vi "GUI_LPG-VikynoRV125.vi"() -> ()   [LabVIEW 2020]
uses:
  <vilib>/Instr/_visa.llb/VISA Configure Serial Port (Instr).vi
panel:
  out "Gen Torque (N.m)":sgl format="%#_6f"
  out "Engine Speed (RPM)":sgl(knob) scale=0.0..2500.0
  out "Average MAF Value (g/s)":dbl format="%.2f"
  in  "Reset Torque":bool
  out "MAF (g/s)":dbl format="%.2f"
  in  "Diesel Used (g)":dbl
  in  "LPG  Consumed (g)":dbl
  out "Engine Torque (N.m)":dbl format="%#_4f"
  out "Equivalent Ratio (Phi)":dbl format="%.2f"
  out "Engine Power (kW)":dbl
  in  "Tab Control":enum32{"PID", "Error"}(tab)
  out "PID Engine Speed Graph":cluster{sgl, "Set Engine Speed":sgl}(graph)
  out "Actual Engine Speed (RPM)":sgl
  out "error out":errorcluster
  out "error out 2":errorcluster
  in  "Stop":bool
  in  "Number of sample":u16=50
  out "?":bool
  out "?":bool
  in  "Arduino UNO port":refnum<visa-resource-name>="COM8"
  in  "Loop Time (ms)":u32=25
  in  "ESP32 port":refnum<visa-resource-name>="COM9"
  in  "INJT 2 (CA)":sgl=10.0 min=0 max=720 format="%#.1f"
  in  "INJT 1 (CA)":sgl=10.0 min=0 max=720 format="%#.1f"
  out "AVG Injection duration (ms)":sgl format="%#.4f"
  in  "?":bool
  out "KI":sgl
  out "KD":sgl
  out "KP":sgl
  in  "LPG Injection":bool
  in  "Set Engine Speed":sgl=1800.0
  out "Injection Duration (ms)":sgl format="%#.4f"
  in  "Kd:":sgl=0.02
  in  "Ki:":sgl=1.2
  in  "Kp:":sgl=0.5
  out "read buffer sensor":string
  out "read buffer ne PID":string
  # "INDUSTRIAL UNIVERSITY OF HO CHI MINH CITY"
  # "Faculty of Automotive Engineering Technology"
  # "Engine Indicators"
  # "Speed Indicator"
  # "Control Panel"
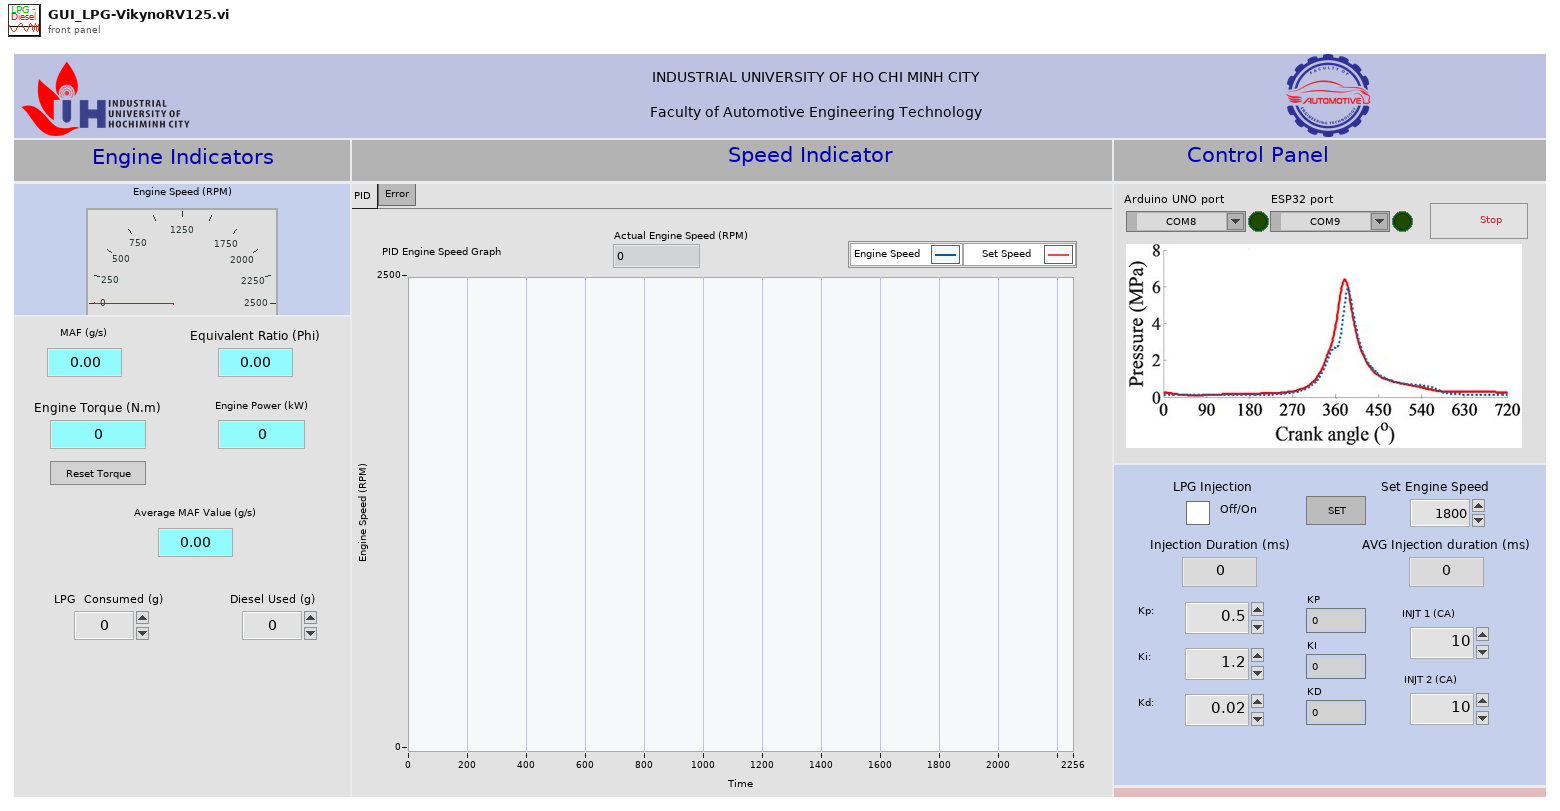
[diagram p1: front panel]
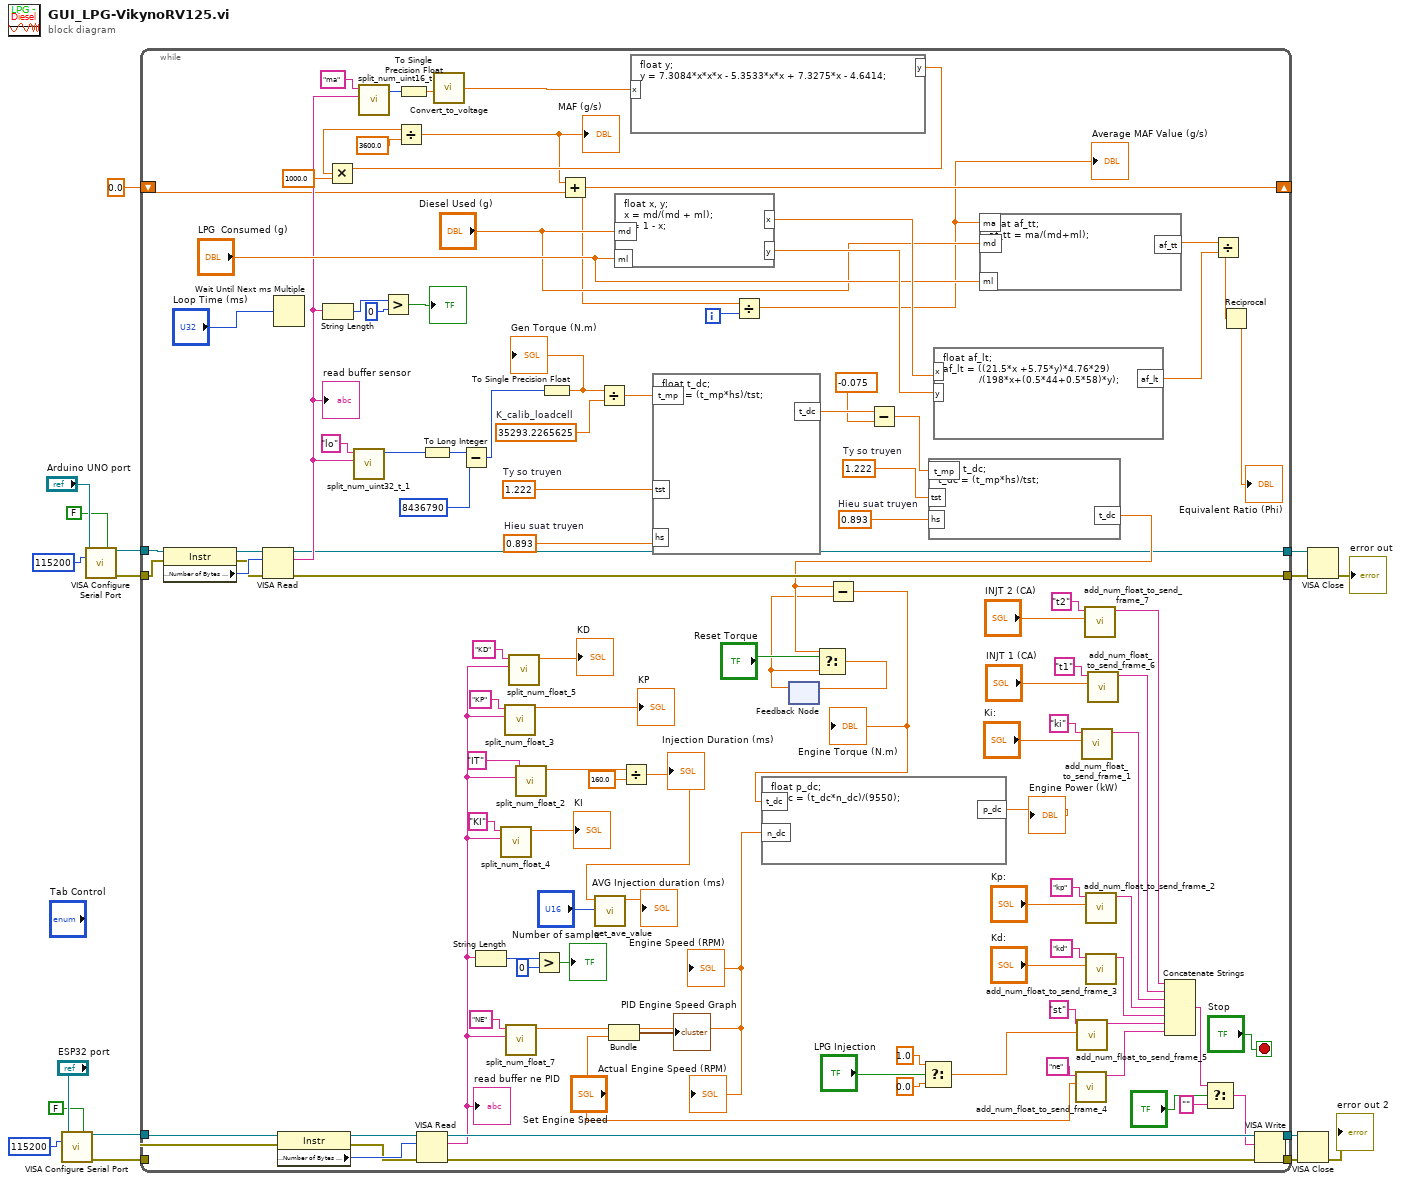
[diagram p0: block diagram]
diagram:
  n1 = call-poly "VISA Configure Serial Port"("VISA resource name"="ESP32 port", "Enable Termination\nChar (T)"=FALSE ("Enable Termination\nChar (T)"), "baud rate (9600)"=u32 115200) -> ("VISA resource name out"=w11:refnum<visa-resource-name>, "error out"=w10:errorcluster)  [unwired: 11 in]
  n2 = call-poly "VISA Configure Serial Port"("VISA resource name"="Arduino UNO port", "Enable Termination\nChar (T)"=FALSE ("Enable Termination\nChar (T)"), "baud rate (9600)"=u32 115200) -> ("VISA resource name out"=w16:refnum<visa-resource-name>, "error out"=w14:errorcluster)  [unwired: 11 in]
  n3 = while {
    tunnel: w16 -> [w127]
    tunnel: [w36] -> w15
    tunnel: w14 -> [w123]
    tunnel: [w121] -> w13
    tunnel: w11 -> [w117]
    tunnel: w10 -> [w116]
    tunnel: [w112] -> w7
    tunnel: [w110] -> w6
    shift-right: [w49] -> _
    shift-left: 0.0 -> [w34]
    i -> [w48]
    stop <- "Stop" stop-if-true
    w58 = 0.893  # Hieu suat truyen
    w59 = 1.222  # Ty so truyen
    w76 = 0.893  # Hieu suat truyen
    w77 = 1.222  # Ty so truyen
    w71 = sgl 35293.227  # K_calib_loadcell
    n4 = property class="Instr"(reference=w127, error in=w123) -> (reference out=w126:refnum<visa-resource-name>, error out=w122:errorcluster, "Serial Settings:Number of Bytes at Serial Port"=w125:u32)
    n5 = VISA Read(VISA resource name=w126, byte count=w125, error in (no error)=w122) -> (VISA resource name out=w36:refnum<visa-resource-name>, read buffer=w68:string, error out=w121:errorcluster)  [unwired: 1 out]
    "read buffer sensor" <- w68
    n6 = Wait Until Next ms Multiple(millisecond multiple="Loop Time (ms)") -> ()  [unwired: 1 out]
    n7 = property class="Instr"(reference=w117, error in=w116) -> (reference out=w120:refnum<visa-resource-name>, error out=w118:errorcluster, "Serial Settings:Number of Bytes at Serial Port"=w119:u32)
    n8 = String Length(string=w68) -> (length=w67:i32)
    n9 = call "split_num_uint32_t_1.vi"("read_frame"=w68, "id (2 characters)"="lo") -> ("num_uint32_t"=w87:u32)  [unwired: 9 in]
    n10 = call "split_num_uint16_t.vi"("read_frame"=w68, "id (2 characters)"="ma") -> ("num_uint16_t"=w43:u16)  [unwired: 9 in]
    n11 = Greater?(x=w67, y=0) -> (0:→"?":bool)
    n12 = To Single Precision Float(number=w43) -> (single precision float=w42:sgl)
    n13 = VISA Read(VISA resource name=w120, byte count=w119, error in (no error)=w118) -> (VISA resource name out=w113:refnum<visa-resource-name>, read buffer=w20:string, error out=w111:errorcluster)  [unwired: 1 out]
    "read buffer ne PID" <- w20
    n14 = To Long Integer(number=w87) -> (32bit integer=w73:i32)
    n15 = call "Convert_to_voltage.vi"("Digital Value"=w42) -> ("Voltage Out"=w46:sgl)  [unwired: 8 in]
    n16 = Subtract(x=w73, y=8436790) -> (x-y=w60:i32)
    n17 = String Length(string=w20) -> (length=w63:i32)
    n18 = call "split_num_float_4.vi"("read_frame"=w20, "id (2 characters)"="KI") -> ("num_float"=→"KI":sgl)  [unwired: 9 in]
    n19 = call "split_num_float_3.vi"("read_frame"=w20, "id (2 characters)"="KP") -> ("num_float"=→"KP":sgl)  [unwired: 9 in]
    n20 = call "split_num_float_7.vi"("read_frame"=w20, "id (2 characters)"="NE") -> ("num_float"=w40:sgl)  [unwired: 9 in]
    "Engine Speed (RPM)" <- w40
    "Actual Engine Speed (RPM)" <- w40
    n21 = call "split_num_float_5.vi"("read_frame"=w20, "id (2 characters)"="KD") -> ("num_float"=→"KD":sgl)  [unwired: 9 in]
    n22 = call "split_num_float_2.vi"("read_frame"=w20, "id (2 characters)"="IT") -> ("num_float"=w18:sgl)  [unwired: 9 in]
    n23 = Greater?(x=w63, y=0) -> (0:→"?":bool)
    n24 = To Single Precision Float(number=w60) -> (single precision float=w61:sgl)
    "Gen Torque (N.m)" <- w61
    n25 = Divide(x=w61, y=w71) -> (x/y=w74:sgl)
    n26 = Bundle("num_float"=w40, "Set Engine Speed"="Set Engine Speed") -> (→"PID Engine Speed Graph":cluster{"num_float":sgl, "Set Engine Speed":sgl})  [unwired: 1 in]
    n27 = formula code="float x, y;\nx = md/(md + ml);\ny = 1 - x;"("md"="Diesel Used (g)", "ml"="LPG  Consumed (g)") -> ("x"=w85:dbl, "y"=w84:dbl)
    n28 = Divide(x=w18, y=sgl 160.0) -> (x/y=w41:sgl)
    "Injection Duration (ms)" <- w41
    n29 = call "get_ave_value.vi"("number_of_values"="Number of sample", "value_in (convert to sgl)"=w41) -> ("ave_value"=→"AVG Injection duration (ms)":sgl)  [unwired: 9 in]
    n30 = formula code="float y;\ny = 7.3084*x*x*x - 5.3533*x*x + 7.3275*x - 4.6414;"("x"=w46) -> ("y"=w99:dbl)
    n31 = Multiply(x=w99, y=1000.0) -> (x*y=w57:dbl)
    n32 = Divide(x=w57, y=3600.0) -> (x/y=w33:dbl)
    "MAF (g/s)" <- w33
    n33 = Add(x=w33, y=w34) -> (x+y=w49:dbl)
    n34 = formula code="float t_dc;\nt_dc = (t_mp*hs)/tst;"("t_mp"=w74, "tst"=w77, "hs"=w76) -> ("t_dc"=w70:dbl)
    n35 = Divide(x=w49, y=w48) -> (x/y=w47:dbl)
    "Average MAF Value (g/s)" <- w47
    n36 = feedback #1() -> (w50:dbl)  [unwired: 1 in]
    n37 = Subtract(x=w70, y=-0.075) -> (x-y=w55:dbl)
    n38 = Select(t=sgl 1.0, s="LPG Injection", f=sgl 0.0) -> (s? t:f=w37:sgl)
    n39 = formula code="float t_dc;\nt_dc = (t_mp*hs)/tst;"("t_mp"=w55, "tst"=w59, "hs"=w58) -> ("t_dc"=w51:dbl)
    n40 = Select(t=w51, s="Reset Torque", f=w50) -> (s? t:f=w53:dbl)
    n41 = feedback-in #1(w53) -> ()
    n42 = Subtract(x=w51, y=w50) -> (x-y=w54:dbl)
    "Engine Torque (N.m)" <- w54
    n43 = formula code="float p_dc;\np_dc = (t_dc*n_dc)/(9550);"("t_dc"=w54, "n_dc"=w40) -> ("p_dc"=→"Engine Power (kW)":dbl)
    n44 = formula code="float af_lt;\naf_lt = ((21.5*x +5.75*y)*4.76*29)\n            /(198*x+(0.5*44+0.5*58)*y);"("x"=w85, "y"=w84) -> ("af_lt"=w82:dbl)
    n45 = formula code="float af_tt;\naf_tt = ma/(md+ml);"("md"="Diesel Used (g)", "ml"="LPG  Consumed (g)", "ma"=w47) -> ("af_tt"=w83:dbl)
    n46 = call "add_num_float_to_send_frame_4.vi"("num_float"="Set Engine Speed", "id (2 characters)"="ne") -> ("String"=w21:string)  [unwired: 9 in]
    n47 = call "add_num_float_to_send_frame_5.vi"("num_float"=w37, "id (2 characters)"="st") -> ("String"=w22:string)  [unwired: 9 in]
    n48 = call "add_num_float_to_send_frame_1.vi"("num_float"="Ki:", "id (2 characters)"="ki") -> ("String"=w25:string)  [unwired: 9 in]
    n49 = call "add_num_float_to_send_frame_7.vi"("num_float"="INJT 2 (CA)", "id (2 characters)"="t2") -> ("String"=w27:string)  [unwired: 9 in]
    n50 = call "add_num_float_to_send_frame_2.vi"("num_float"="Kp:", "id (2 characters)"="kp") -> ("String"=w24:string)  [unwired: 9 in]
    n51 = call "add_num_float_to_send_frame_3.vi"("num_float"="Kd:", "id (2 characters)"="kd") -> ("String"=w23:string)  [unwired: 9 in]
    n52 = call "add_num_float_to_send_frame_6.vi"("num_float"="INJT 1 (CA)", "id (2 characters)"="t1") -> ("String"=w26:string)  [unwired: 9 in]
    n53 = Concatenate Strings(w27, w26, w25, w24, w23, w22, w21) -> (w28:string)
    n54 = Select(t=w28, s="?", f="") -> (s? t:f=w91:string)
    n55 = Divide(x=w83, y=w82) -> (x/y=w79:dbl)
    n56 = Reciprocal(x=w79) -> (1/x=→"Equivalent Ratio (Phi)":dbl)
    n57 = VISA Write(VISA resource name=w113, write buffer=w91, error in (no error)=w111) -> (VISA resource name out=w112:refnum<visa-resource-name>, error out=w110:errorcluster)  [unwired: 1 out]
  }
  n58 = VISA Close(VISA resource name=w7, error in (no error)=w6) -> (error out=→"error out 2":errorcluster)
  n59 = VISA Close(VISA resource name=w15, error in (no error)=w13) -> (error out=→"error out":errorcluster)
